vi "PM100D_Close.vi"(1 "Mode":T1=2 items=["Deassert REN", "Assert REN", "Go To Local; Deassert REN ", "Assert REN; Address Device", "Local Lockout (Addressed Devices)", "Local Lockout (This Device)", "Go To Local"], 2 "error in (no error)":errorcluster, 3 "VISA resource name":refnum<visa-resource-name>) -> ()   [LabVIEW 2011]
doc: "Closes the VISA session\nSets the connected instrument in local mode (default option)"
uses:
  <vilib>/Instr/_visa.llb/VISA GPIB Control REN Mode.ctl
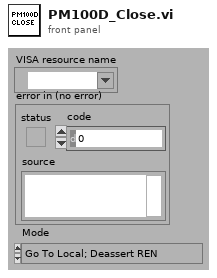
[diagram p1: front panel]
types:
  T1 = typedef "VISA GPIB Control REN Mode.ctl" = u16
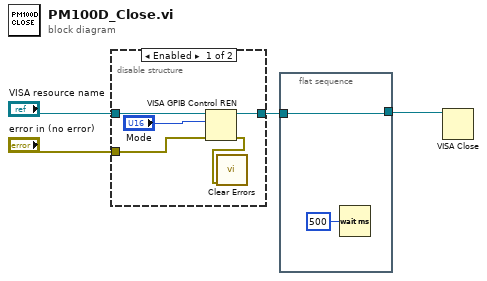
[diagram p0: block diagram]
diagram:
  n1 = disable-structure shown="Enabled" {
    disable-tunnel: "VISA resource name" -> [w8 _]
    disable-tunnel: "error in (no error)" -> [w7 _]
    disable-tunnel: [w6 _] -> w2
    frame Enabled {
      n2 = VISA GPIB Control REN(8:w7, 10:"Mode", 11:w8) -> (0:w5:errorcluster, 3:w6:refnum<visa-resource-name>)
      n3 = call <vilib>:"Clear Errors.vi"("error in (no error)"=w5) -> ()  [unwired: 6 in, 1 out]
    }
    frame Disabled {
    }
  }
  n4 = flat-sequence {
    tunnel: [w11] -> w1
    tunnel: w2 -> [w11]
    frame #0 {
      n5 = Wait (ms)(milliseconds to wait=u32 500) -> ()  [unwired: 1 out]
    }
  }
  n6 = VISA Close(VISA resource name=w1) -> ()  [unwired: 1 in, 1 out]
